vi "test_riccat_03Ni.vi"() -> (3 "All Tests Passed":bool)   [LabVIEW 2019]
uses:
  <vilib>/Analysis/Matrix/Datatypes/RealMatrix.ctl
  <vilib>/Rock Robotics/WPI/ThirdParty/JAS_Junk/TrajLib/Trajectory_Library.lvlib
  <vilib>/Analysis/Matrix/NI_Matrix.lvlib
panel:
  out "R1":T1
  out "Q1":T1
  out "N1":T1
  out "Make QRN Good":bool
  in  "AREF":T1=[[0.0, 0.5], [0.0, 0.0]]
  out "error out 2":errorcluster
  out "Pos Semi Definite":bool
  out "Q_Chk_Passed":bool
  out "C":T1
  out "Q Check":T1
  out "Bad":bool
  out "Stable Bad":bool
  out "error out":errorcluster
  out "Eigenvalues":cdb[](array[numeric])
  out "Error":bool
  out "Iterations":i32
  out "Elapsed \nTime MS":dbl
  out "ZERO":T1
  out "X  Answer":T1
  in  "R":T1=[[1.0]]
  in  "Q":T1=[[1.0, 0.0], [0.0, 1.0]]
  in  "B":T1=[[0.0], [1.0]]
  in  "A":T1=[[0.0, 1.0], [0.0, 0.0]]
  # "// Test 3: the first generalized eigenvalue of (S,T) is stable"
  # "A3 << \n           0, 1, \n           0, 0;"
  # "B3 << \n0, \n1;"
  # "Q3 << \n      1, 0,\n      0, 1;"
  # "Example G2"
  # "Cost ??"
  # "R3 << 1;"
  # "0, 0.5, \n0, 0"
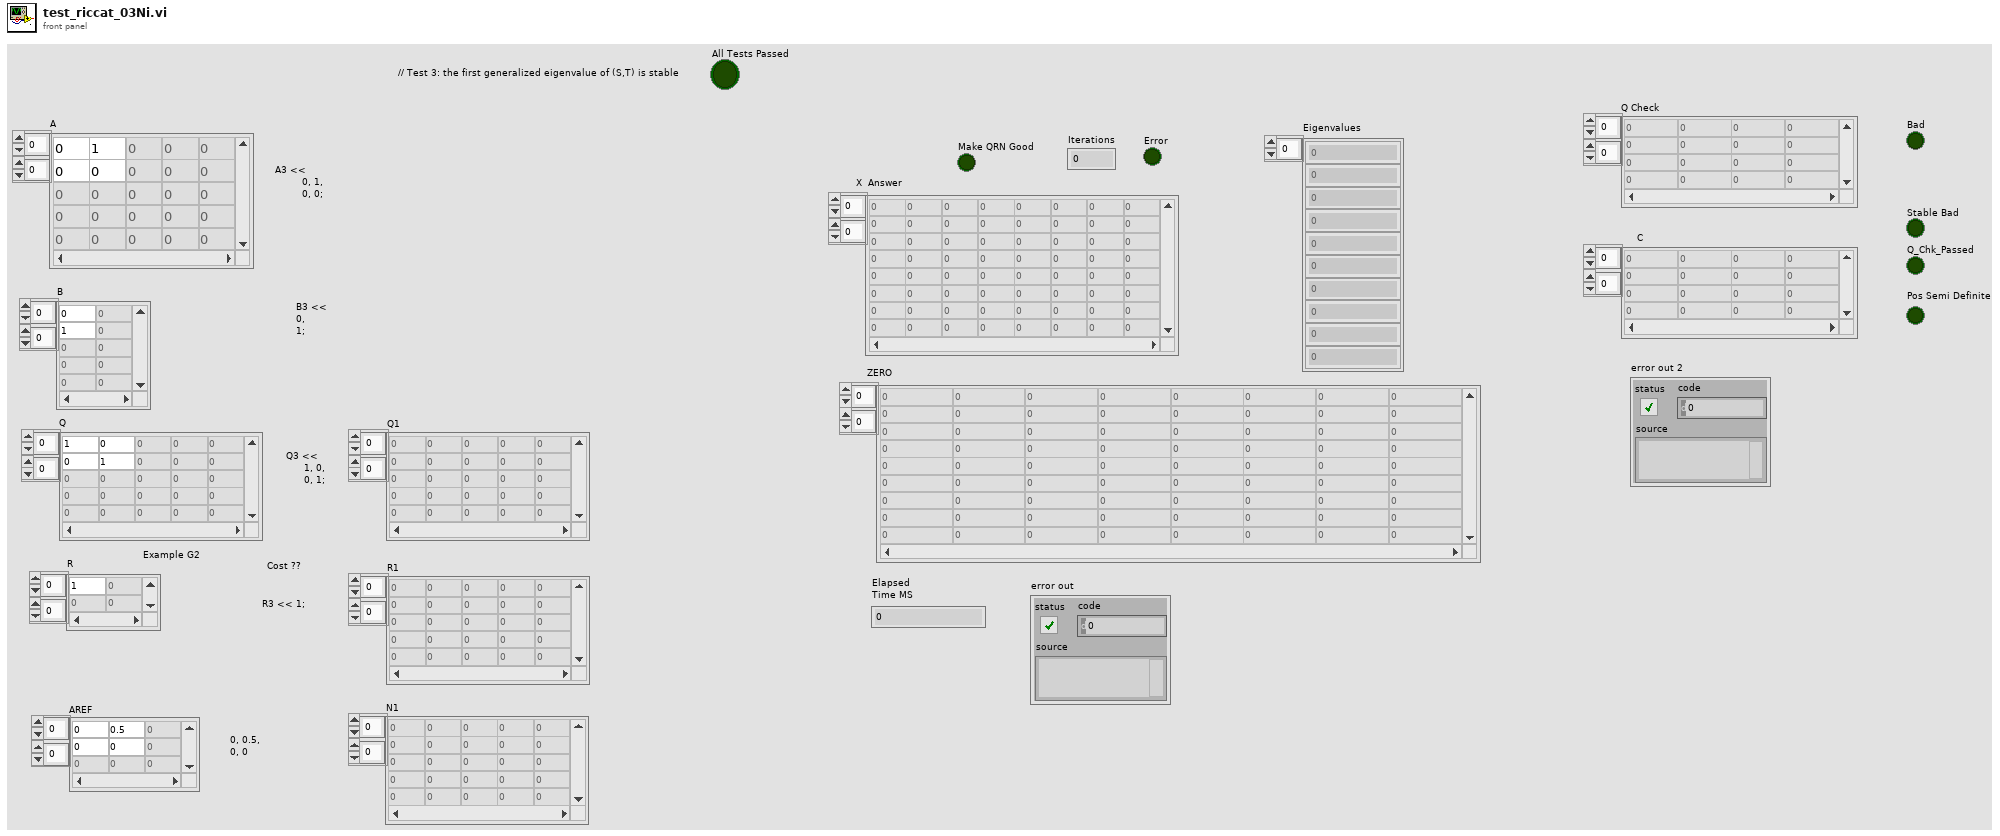
[diagram p1: front panel]
types:
  T1 = typedef "NI_Matrix.lvlib/RealMatrix.ctl" = dbl[][]
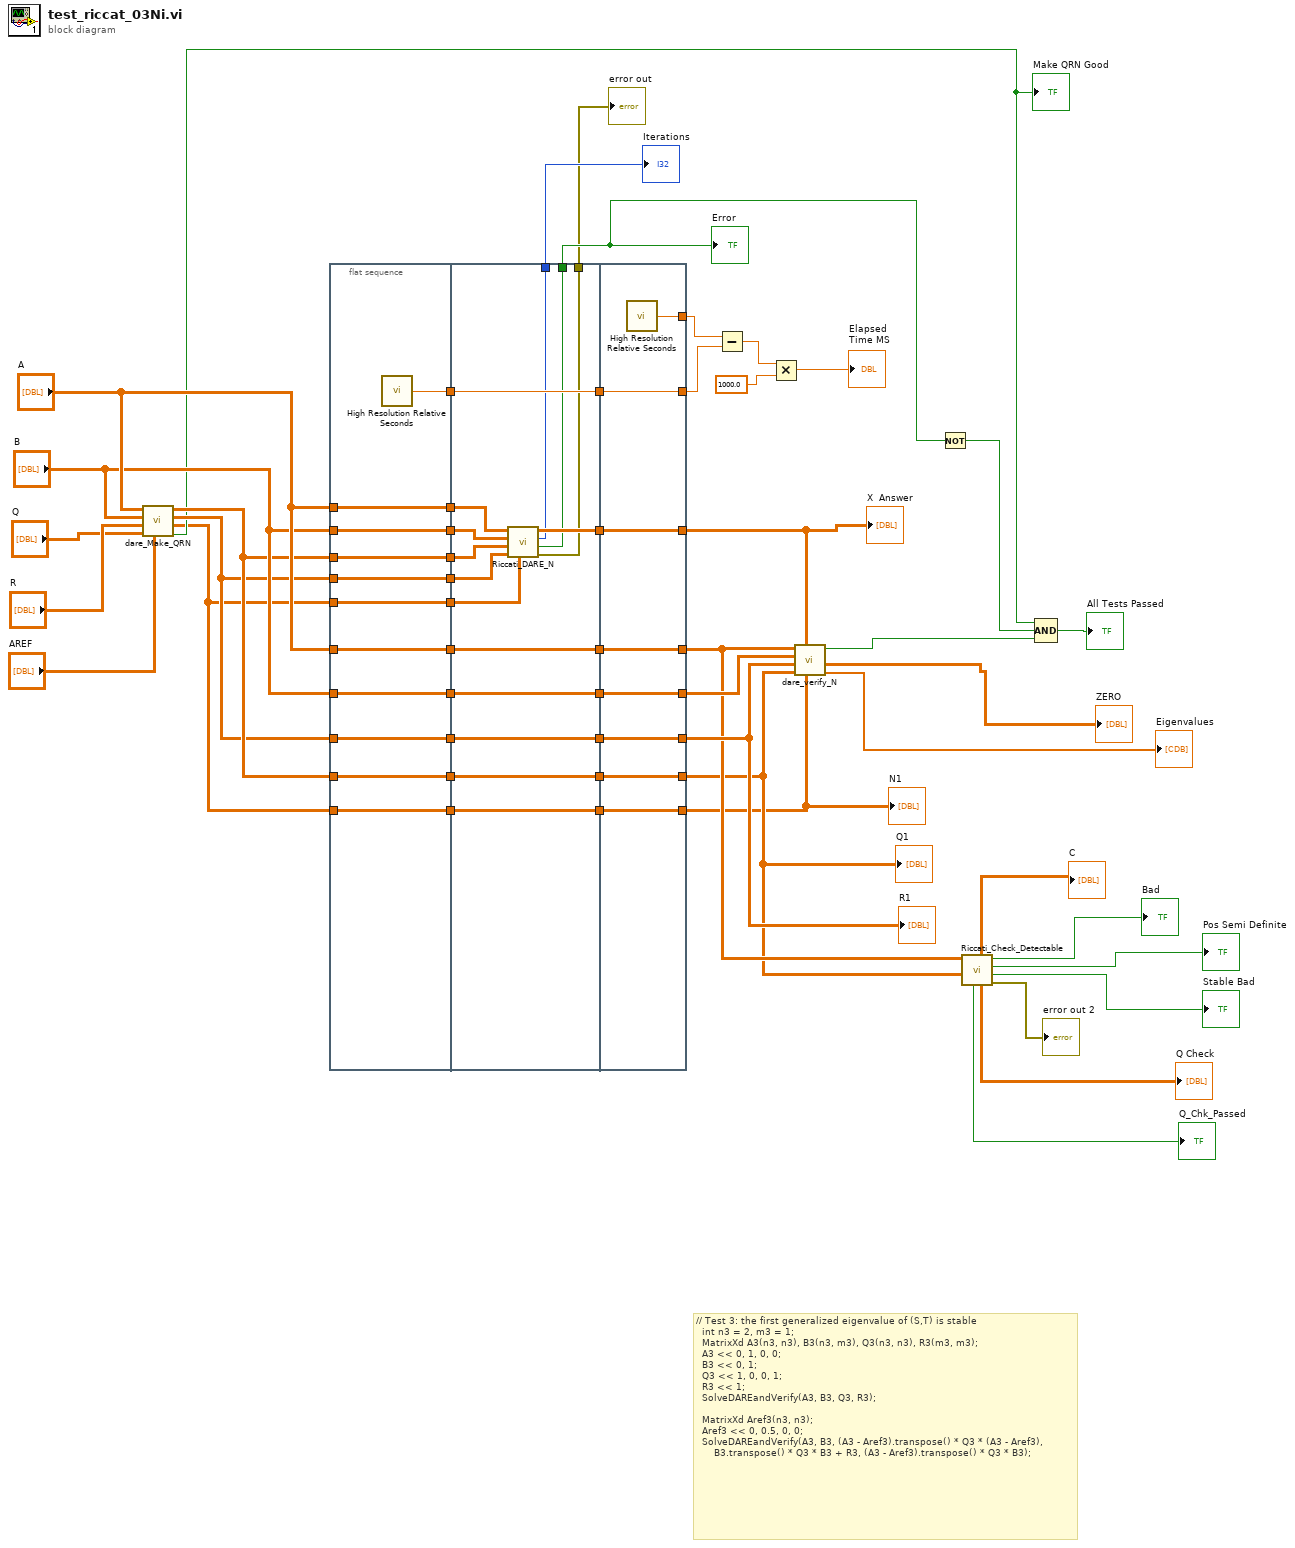
[diagram p0: block diagram]
diagram:
  # "// Test 3: the first generalized eigenvalue of (S,T) is stable\n  int n3 = 2, m3 = 1;\n  MatrixXd A3(n3, n3), B3(n3, m3), Q3(n3, n3), R3(m3, m3);\n  A3 << 0, 1, 0, 0;\n  B3 << 0, 1;\n  Q3 << 1, 0, 0, 1;\n  R3 << 1;\n  SolveDAREandVerify(A3, B3, Q3, R3);\n\n  MatrixXd Aref3(n3, n3);\n  Aref3 << 0, 0.5, 0, 0;\n  SolveDAREandVerify(A3, B3, (A3 - Aref3).transpose() * Q3 * (A3 - Aref3),\n      B3.transpose() * Q3 * B3 + R3, (A3 - Aref3).transpose() * Q3 * B3);"
  n1 = call "dare_Make_QRN.vi"("AREF"="AREF", "Q"="Q", "R"="R", "B"="B", "A"="A") -> ("Good"=w5:bool, "N1"=w4:T1, "R1"=w7:T1, "Q1"=w8:T1)  [unwired: 3 in]
  "Make QRN Good" <- w5
  n2 = flat-sequence {
    tunnel: "B" -> [w59]
    tunnel: "A" -> [w60]
    tunnel: "B" -> [w61]
    tunnel: w8 -> [w62]
    tunnel: "A" -> [w63]
    tunnel: w7 -> [w64]
    tunnel: [w64] -> w53
    tunnel: [w63] -> w52
    tunnel: [w62] -> w51
    tunnel: [w61] -> w50
    tunnel: [w60] -> w49
    tunnel: [w59] -> w48
    tunnel: w7 -> [w58]
    tunnel: [w58] -> w43
    tunnel: w8 -> [w57]
    tunnel: [w57] -> w42
    tunnel: [w56] -> w37
    tunnel: [w55] -> w6
    tunnel: w4 -> [w55]
    tunnel: w4 -> [w54]
    tunnel: [w54] -> w1
    tunnel: w53 -> [w79]
    tunnel: w52 -> [w77]
    tunnel: w51 -> [w76]
    tunnel: w50 -> [w75]
    tunnel: w49 -> [w74]
    tunnel: w48 -> [w73]
    tunnel: [w78] -> w47
    tunnel: [w74] -> w46
    tunnel: [w73] -> w45
    tunnel: [w72] -> w44
    tunnel: w43 -> [w72]
    tunnel: w42 -> [w71]
    tunnel: [w71] -> w41
    tunnel: [w70] -> w38
    tunnel: w37 -> [w70]
    tunnel: [w69] -> w33
    tunnel: [w68] -> w27
    tunnel: [w67] -> w23
    tunnel: w6 -> [w66]
    tunnel: [w65] -> w2
    tunnel: w1 -> [w65]
    tunnel: [w85] -> w31
    tunnel: [w86] -> w20
    tunnel: [w87] -> w32
    tunnel: w47 -> [w87]
    tunnel: w46 -> [w86]
    tunnel: w45 -> [w85]
    tunnel: [w84] -> w30
    tunnel: w44 -> [w84]
    tunnel: [w83] -> w19
    tunnel: w41 -> [w83]
    tunnel: [w82] -> w40
    tunnel: [w81] -> w39
    tunnel: w38 -> [w81]
    tunnel: [w80] -> w3
    tunnel: w2 -> [w80]
    frame #0 {
      n3 = call <vilib>:"High Resolution Relative Seconds.vi"() -> ("relative seconds"=w56:dbl)
    }
    frame #1 {
      n4 = call <vilib>:"Riccati_DARE_N.vi"("N"=w66, "R"=w79, "Q"=w76, "B"=w75, "A"=w77) -> ("error out"=w67:errorcluster, "Error"=w68:bool, "Iterations"=w69:i32, "Answer"=w78:T1)  [unwired: 3 in]
    }
    frame #2 {
      n5 = call <vilib>:"High Resolution Relative Seconds.vi"() -> ("relative seconds"=w82:dbl)
    }
  }
  n6 = Subtract(x=w40, y=w39) -> (x-y=w36:dbl)
  n7 = Multiply(x=w36, y=1000.0) -> (x*y=→"Elapsed \nTime MS":dbl)
  n8 = call "dare_verify_N.vi"("N"=w3, "Answer"=w32, "Q"=w19, "R"=w30, "B"=w31, "A"=w20) -> ("Eigenvalues"=→"Eigenvalues":cdb[], "ZERO"=→"ZERO":T1, "Passed"=w28:bool)  [unwired: 3 in]
  n9 = Not(x=w27) -> (.not. x?=w26:bool)
  n10 = call <vilib>:"Riccati_Check_Detectable.vi"("Q"=w19, "A"=w20) -> ("error out"=→"error out 2":errorcluster, "Stable Bad"=→"Stable Bad":bool, "Pos Semi Definite"=→"Pos Semi Definite":bool, "Bad"=→"Bad":bool, "Q_Check"=→"Q Check":T1, "C"=→"C":T1, "Q_Chk_Passed"=→"Q_Chk_Passed":bool)  [unwired: 3 in]
  n11 = Compound Arithmetic op=AND(w5, w26, w28) -> (→"All Tests Passed":bool)
  "X  Answer" <- w32
  "Iterations" <- w33
  "Error" <- w27
  "error out" <- w23
  "N1" <- w3
  "Q1" <- w19
  "R1" <- w30
